vi "Initialize Initializing.vi"(10 "output cluster":T1, 11 "path":path) -> ()   [LabVIEW 2016]
uses:
  Controls/Cal Refs.ctl
  Miscellaneous/Globals.vi
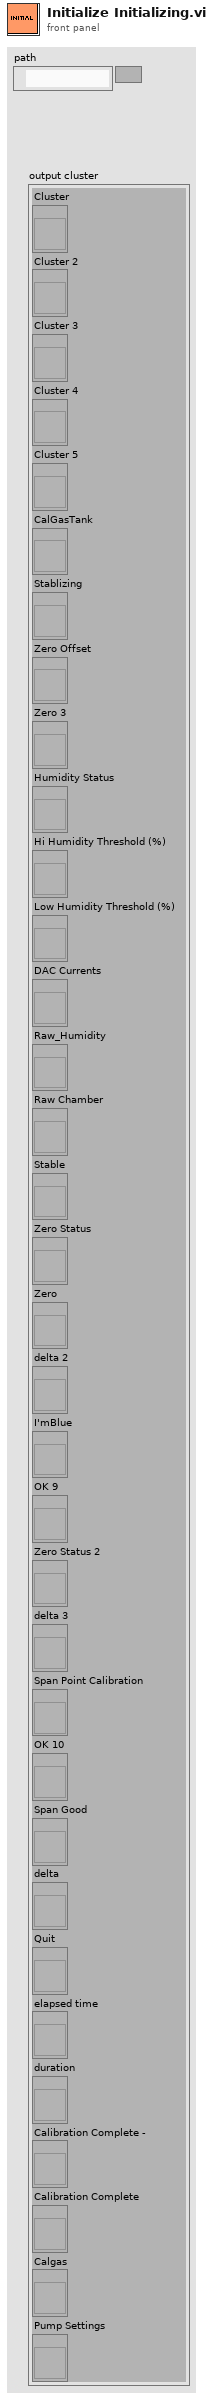
[diagram p1: front panel]
types:
  T1 = typedef "Cal Refs.ctl" = cluster{"Cluster":refnum<vi>, "Cluster 2":refnum<vi>, "Cluster 3":refnum<vi>, "Cluster 4":refnum<vi>, "Cluster 5":refnum<vi>, "CalGasTank":refnum<vi>, "Stablizing":refnum<vi>, "Zero Offset":refnum<vi>, "Zero 3":refnum<vi>, "Humidity Status":refnum<vi>, "Hi Humidity Threshold (%)":refnum<vi>, "Low Humidity Threshold (%)":refnum<vi>, "DAC Currents":refnum<vi>, "Raw_Humidity":refnum<vi>, "Raw Chamber":refnum<vi>, "Stable":refnum<vi>, "Zero Status":refnum<vi>, "Zero":refnum<vi>, "delta 2":refnum<vi>, "I'mBlue":refnum<vi>, "OK 9":refnum<vi>, "Zero Status 2":refnum<vi>, "delta 3":refnum<vi>, "Span Point Calibration":refnum<vi>, "OK 10":refnum<vi>, "Span Good":refnum<vi>, "delta":refnum<vi>, "Quit":refnum<vi>, "elapsed time":refnum<vi>, "duration":refnum<vi>, "Calibration Complete -":refnum<vi>, "Calibration Complete":refnum<vi>, "Calgas":refnum<vi>, "Pump Settings":refnum<vi>}
  T2 = enum32{"Invalid", "Standard", "Closed", "Hidden", "Minimized", "Maximized"}
  T3 = typedef "Pump Settings.ctl" = cluster{"Flow":u16, "Solenoid#1":bool, "Solenoid#2":bool, "ignore":bool}
  T4 = cluster{"Tcal_Chamber":dbl, "Tcal_PCB":dbl, "Tcal_Film":dbl, "Tcal_Humidity":dbl, "Tcal_Det":dbl[], "Cal Gas":dbl, "Reference":dbl}
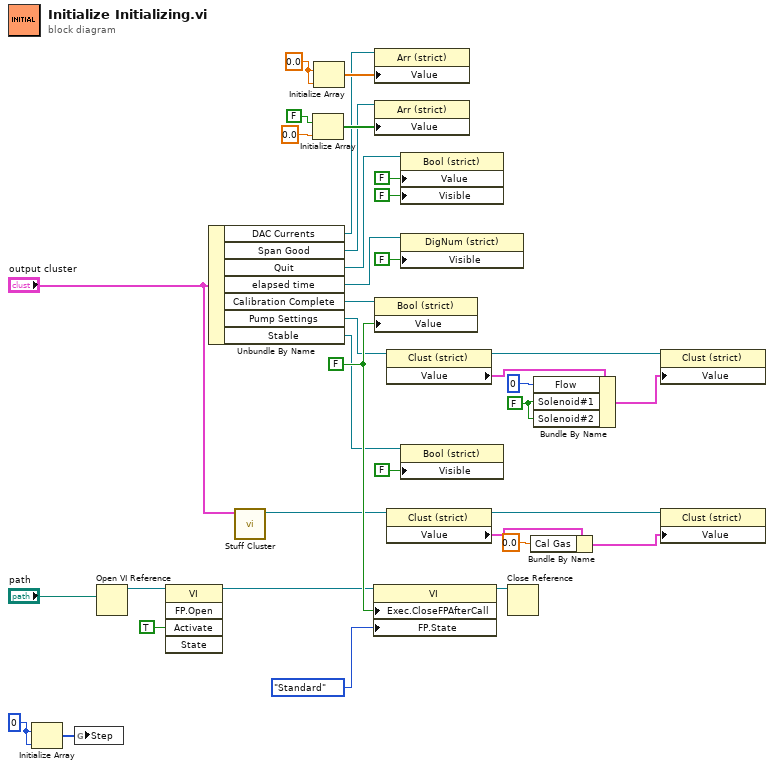
[diagram p0: block diagram]
diagram:
  w4 = FALSE
  w17 = 0.0
  w16 = 0
  w35 = FALSE ("Calibration Complete")
  n1 = Initialize Array(w16, w16) -> (w24:i32[])
  n2 = global write "Globals.vi" "Step"(w24) -> ()
  n3 = Open VI Reference(vi path="path") -> (vi reference=w12:refnum<vi>)  [unwired: 5 in, 1 out]
  n4 = invoke class="VI" method="FP.Open"(reference=w12, "Activate"=TRUE ("Activate?")) -> (reference out=w11:refnum<vi>)  [unwired: 3 in, 4 out]
  n5 = Unbundle By Name("output cluster") -> ("DAC Currents"=w25:refnum<vi>, "Span Good"=w28:refnum<vi>, "Quit"=w30:refnum<vi>, "elapsed time"=w33:refnum<vi>, "Calibration Complete"=w34:refnum<vi>, "Pump Settings"=w9:refnum<vi>, "Stable"=w3:refnum<vi>)
  n6 = call "Stuff Cluster.vi"("output cluster"="output cluster") -> ("reference out"=w27:refnum<vi>)  [unwired: 10 in]
  n7 = Initialize Array(FALSE, 0.0) -> (w29:bool[])
  n8 = Initialize Array(w17, w17) -> (w36:dbl[])
  n9 = property class="VI"(reference=w11, "Exec.CloseFPAfterCall"=w35, "FP.State"=T2."Standard" ("Front Panel Window:State")) -> (reference out=w13:refnum<vi>)  [unwired: 1 in, 1 out]
  n10 = property class="Arr (strict)"(reference=w25, "Value"=w36) -> ()  [unwired: 1 in, 2 out]
  n11 = property class="Arr (strict)"(reference=w28, "Value"=w29) -> ()  [unwired: 1 in, 2 out]
  n12 = property class="Bool (strict)"(reference=w34, "Value"=w35) -> ()  [unwired: 1 in, 2 out]
  n13 = property class="Clust (strict)"(reference=w9) -> (reference out=w8:refnum<vi>, "Value"=w7:T3)  [unwired: 1 in, 1 out]
  n14 = property class="Clust (strict)"(reference=w27) -> (reference out=w20:refnum<vi>, "Value"=w21:T4)  [unwired: 1 in, 1 out]
  n15 = property class="Bool (strict)"(reference=w30, "Value"=FALSE ("Cal Fail"), "Visible"=FALSE ("Blinking")) -> ()  [unwired: 1 in, 2 out]
  n16 = property on="Property Node" class="DigNum (strict)"(reference=w33, "Visible"=FALSE) -> ()  [unwired: 1 in, 2 out]
  n17 = property on="Property Node" class="Bool (strict)"(reference=w3, "Visible"=FALSE) -> ()  [unwired: 1 in, 2 out]
  n18 = Close Reference(reference=w13) -> ()  [unwired: 1 in, 1 out]
  n19 = Bundle By Name(cluster=w21, "Cal Gas"=0.0) -> (w22:T4)
  n20 = Bundle By Name(cluster=w7, "Flow"=u16 0, "Solenoid#1"=w4, "Solenoid#2"=w4) -> (w6:T3)
  n21 = property class="Clust (strict)"(reference=w8, "Value"=w6) -> ()  [unwired: 1 in, 2 out]
  n22 = property class="Clust (strict)"(reference=w20, "Value"=w22) -> ()  [unwired: 1 in, 2 out]
